vi "ASE Kalman_Experiment_FPGA.vi"() -> ()   [LabVIEW 2018]
doc: "This example demonstrates a simple analog loopback."
uses:
  <vilib>/Simulation/Scripting/Companion Diagram/SimConfigNode/SimParams.ctl
  <vilib>/Simulation/Scripting/Companion Diagram/SimConfigNode/_simSolvers.ctl
  <vilib>/Simulation/Implementation/Shared/SIMSCR Execution Mode.ctl
  <vilib>/Platform/TimedLoop/XDataNode/timing_clust.ctl
  <vilib>/Platform/TimedLoop/XDataNode/nitl_modes.ctl
  <vilib>/Platform/TimedLoop/XDataNode/wakeup.ctl
  <vilib>/Simulation/Param Hierarchy/Typedefs/SIMPH Param Control Actions.ctl
  <vilib>/addons/Control Design/_Stochastic Systems/Stochastic Systems.llb/Stochastic Systems SubVIs/cd_Second-Order Statistics Noise Model.ctl
  <vilib>/Simulation/Implementation/Shared/SIM limit type.ctl
  <vilib>/Simulation/Scripting/Editor Utilities/SIM subVI tag data.ctl
  <vilib>/Simulation/Scripting/Editor Utilities/SIM subVI execution type.ctl
  <vilib>/Simulation/Implementation/Shared/NILVSim_ParamChanged.vi
  <vilib>/Simulation/Implementation/Shared/NILVSim_FinishedLate.vi
  <vilib>/Simulation/Implementation/Shared/NILVSIM_BeginStep.vi
  <vilib>/Simulation/Utility/Implementation/SIM Halt.vi
  <vilib>/Simulation/DataSources/Implementation/NILVSim Signal Generator.llb/SIM Signal Generator (scalar).vi
  <vilib>/Simulation/Nonlinear/Implementation/NILVSim Saturation.llb/SIM Saturation (scalar).vi
  <vilib>/Simulation/ContinuousLinear/Implementation/NILVSim Integrator new.llb/SIM Integrator distributor (scalar).vi
  <vilib>/Simulation/ContinuousLinear/Implementation/NILVSim Integrator new.llb/SIM Integrator collector (scalar).vi
  <vilib>/Simulation/Utility/Implementation/NILVSim Memory.llb/NILVSim Memory (core).vi
  <vilib>/Simulation/ContinuousLinear/Implementation/NILVSim Transfer Function.llb/SIM Transfer Function Distributor (SISO).vi
  <vilib>/Simulation/SignalArithmetic/Implementation/NILVSim Gain.llb/SIM Gain (scalar).vi
  <vilib>/Simulation/ContinuousLinear/Implementation/NILVSim Transfer Function.llb/SIM Transfer Function Collector (SISO).vi
  <vilib>/Simulation/Nonlinear/Implementation/NILVSim RateLimiter.llb/SIM RateLimiter (scalar).vi
  <vilib>/Simulation/Implementation/Shared/SIM Fire Discrete SubVI.vi
  <vilib>/Simulation/Nonlinear/Implementation/NILVSim Saturation.llb/SIM Saturation (vector).vi
  <vilib>/Simulation/SignalArithmetic/Implementation/NILVSim Gain.llb/SIM Gain (vector).vi
  <vilib>/Simulation/SignalDisplay/Implementation/NILVSim Time Waveform.llb/SIM Time Waveform (vector).vi
  <vilib>/Simulation/Implementation/Shared/NILVSim_Manager.vi
  <vilib>/Utility/error.llb/Clear Errors.vi
  <vilib>/Simulation/Implementation/Shared/NILVSim_FinalizeModel.vi
  <vilib>/Simulation/Implementation/Shared/SIM Fire Discrete SubVI (Core).vi
  <vilib>/FPGAPlugInAG/cRIO-9068/niLvFpga_Open_cRIO-9068.vi
  <vilib>/rvi/interface/common/dynamic/niFpgaDynamicAddResources.vi
  <vilib>/imath/engines/lvmath2/RunTimeEngine/Managers/WorkSpace/UID Generator.vi
  <vilib>/imath/engines/lvmath2/RunTimeEngine/RunTimeType/NIMS_RunTimeType_From StrictType (excl LVString).vi
  <instcachedir>/0/NIMS_RunTimeType_From StrictType (excl LVString)_E7E34A65C99947108168652BAD14964D.lvgen/NIMS_RunTimeType_From StrictType (excl LVString)_E7E34A65C99947108168652BAD14964D_000.vi
  <vilib>/imath/engines/lvmath2/RunTimeEngine/LocalVariableDefStatement/MC_LocalVariableDefStatement_Display.vi
  <vilib>/imath/engines/lvmath2/RunTimeEngine/Managers/SymbolTable/Clear UID.vi
  <vilib>/imath/engines/lvmath2/RunTimeEngine/NodeEndStatement/NIMS_NodeEndStatement_Output.vi
  <instcachedir>/0/NIMS_NodeEndStatement_Output_53EC0D466D134D7ABD903AC30B43404B.lvgen/NIMS_NodeEndStatement_Output_53EC0D466D134D7ABD903AC30B43404B_010.vi
  <instcachedir>/0/NIMS_NodeEndStatement_Output_53EC0D466D134D7ABD903AC30B43404B.lvgen/NIMS_NodeEndStatement_Output_53EC0D466D134D7ABD903AC30B43404B_002.vi
  <vilib>/imath/engines/lvmath2/RunTimeEngine/ErrorHandling/NIMS_Finalize Error.vi
  <vilib>/addons/Control Design/_Stochastic Systems/Stochastic Systems.llb/CD Construct Stochastic Model (Numeric).vi
  <vilib>/addons/Control Design/_Stochastic Systems/Stochastic Systems.llb/CD Construct Noise Model (Numeric).vi
  <vilib>/Simulation/Implementation/Shared/SIM Unbundle Sim Info.vi
  <vilib>/Simulation/Implementation/Shared/SIMSH Read Queue.vi
  <vilib>/Simulation/Implementation/Shared/NILVSim_Initialize.vi
  <vilib>/Utility/error.llb/Error Cluster From Error Code.vi
  <vilib>/rvi/errors/niLvFpgaAdjustHostInterfaceError.vi
  <vilib>/Simulation/Utility/Implementation/NILVSim Get Time and IsAcceptedStep.vi
  <vilib>/Simulation/Implementation/Shared/NILVSim_GetModelError.vi
  <vilib>/Simulation/Implementation/Shared/SIM Bundle Sim Info.vi
  <vilib>/FPGAPlugInAG/Dynamic/niLvFpga_Close_Dynamic.vi
  <vilib>/rvi/interface/nirviOpenFPGA/nirviOpenFPGA.xnode
  FPGA Bitfiles/KalmanFilterASE_FPGATarget_FPGAQ1MODULE_8J-A6gSqyPk.lvbitx
  FPGA_Q1_MODULE.vi
  <vilib>/Simulation/Scripting/Companion Diagram/SimConfigNode/SimDog.xnode
  <vilib>/Quanser/Rapid Control Prototyping Toolkit/discrete/_TypeSpecific/CL Bias Removal (Scalar).vi
  <vilib>/Quanser/Rapid Control Prototyping Toolkit/discrete/CL Bias Removal.vi
  <vilib>/addons/Control Design/_Implementation/CD Continuous Recursive Kalman Filter.vi
  <vilib>/Platform/TimedLoop/XDataNode/XDataNode.xnode
  <vilib>/rvi/interface/nirviReadWriteControl/nirviReadWriteControl.xnode
  <vilib>/Simulation/Implementation/XNodeFramework/SimXNode/SimX.xnode
  <vilib>/rvi/interface/nirviCloseFPGA/nirviCloseFPGA.xnode
  <vilib>/Simulation/ContinuousLinear/Implementation/NILVSim Transfer Function.llb/SIM Transfer Function (SISO).vi
  <vilib>/Simulation/ContinuousLinear/Implementation/NILVSim Integrator new.llb/SIM Integrator (scalar).vi
  NiFpgaLv.dll
  <vilib>/rvi/interface/Simulation/niFpgaSimulationCallBeginRW.vi
  <vilib>/addons/Control Design/_Stochastic Systems/NI_CD_Stochastic Systems.lvlib
  <vilib>/imath/engines/lvmath2/RunTimeEngine/Managers/SymbolTable/NIMS_WorkSpace.lvlib
  <vilib>/Platform/TimedLoop/XDataNode/XDNodeRunTimeDep.lvlib
  <vilib>/Simulation/Implementation/Shared/NI_SIM_Implementation.lvlib
panel:
  out "Kalman Filter":waveform(dbl)[](graph)=[{"t0"=timestamp(9.964 s since 1904-01-01), "dt"=1.0, "Y"=[0.009999999999999988]}, {"t0"=timestamp(9.964 s since 1904-01-01), "dt"=1.0, "Y"=[0.008101035650175014]}, {"t0"=timestamp(9.964 s since 1904-01-01), "dt"=1.0, "Y"=[0.0033426903430059957]}]
  out "Measured value":T1(graph)={"output"=0.0096065956, "Result"=0.0090666584, "output"=0.0091514816}
  in  "R":dbl[][](array[numeric])=[[0.001, 0.0], [0.0, 0.001]] format="%#.5f"
  in  "Q":dbl[][](array[numeric])=[[0.001, 0.0, 0.0, 0.0], [0.0, 0.001, 0.0, 0.0], [0.0, 0.0, 0.001, 0.0], [0.0, 0.0, 0.0, 0.001]] format="%#.4f"
  in  "Enable Motor":bool
  in  "Setpoint Command":T2={"Amplitude (m)"=0.01, "Frequency (Hz)"=0.3} caption="Road (Bottom Plate)\nAmplitude Command (m)" {"Frequency (Hz)" min=0.0 max=0.5 step=0.009999999776482582 format="%_3f"; "Amplitude (m)" min=-10.0 max=10.0 step=0.5 format="%_3f"}
  in  "Halt?":bool
  # "Active Suspension Adaptive Control Experiment"
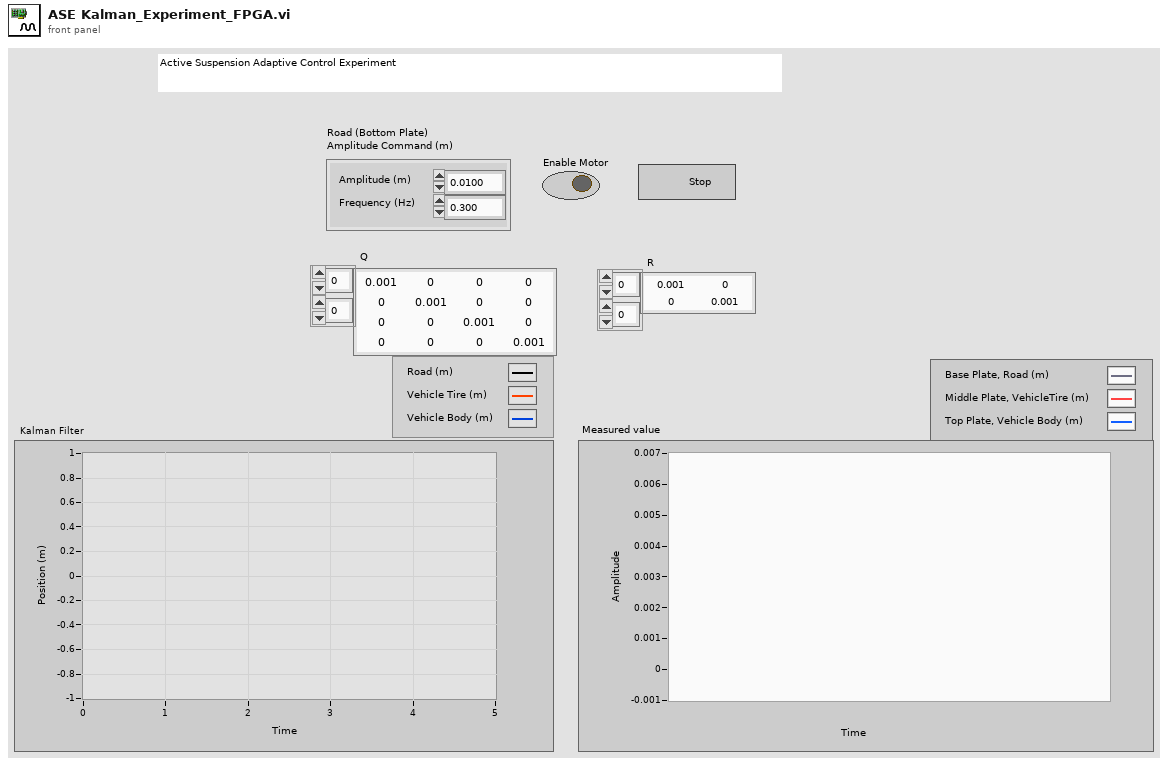
[diagram p1: front panel]
types:
  T1 = cluster{"output":dbl, "Result":dbl, "output":dbl}
  T2 = cluster{"Amplitude (m)":dbl, "Frequency (Hz)":dbl}
  T3 = typedef "SIMSCR Execution Mode.ctl" = enum16{"Simulate to Completion", "Single Time-Step Simulation (Fixed Step Only)"}
  T4 = typedef "XDNodeRunTimeDep.lvlib/timing_clust.ctl" = cluster{"Expected End [f-1]":u64, "Actual End [f-1]":u64, "Finished Late? [f-1]":bool, "Expected End [i-1]":u64, "Actual End [i-1]":u64, "Finished Late? [i-1]":bool, "Expected Start [i]":u64, "Actual Start [i]":u64, "Expected Start [f]":u64, "Actual Start [f]":u64, "Source Name":string, "Structure Name":string, "Period":i64, "Deadline":i64, "Offset":i64, "Start":i64, "Priority":i32, "Timeout":i32, "Mode":T5, "Wakeup Reason":T6, "Error":errorcluster, "Source Type":string, "Secondary Source Type":string, "Global End Time":u64, "Global Start Time":u64, "Frame Duration":u64, "Iteration Duration":u64, "Assigned CPU":i32, "I/O Scan Engine Mode":u32}
  T5 = typedef "XDNodeRunTimeDep.lvlib/nitl_modes.ctl" = enum32{"No Change", "Process missed periods, maintain original phase", "Discard missed periods, maintain original phase", "Process missed periods, ignore original phase", "Discard missed periods, ignore original phase"}
  T6 = typedef "XDNodeRunTimeDep.lvlib/wakeup.ctl" = enum32{"Normal", "Aborted", "Asynchronous wakeup", "Timing source error", "Timed loop error", "Timeout"}
  T7 = typedef "SIMPH Param Control Actions.ctl" = enum16{"get params", "set params"}
  T8 = typedef "SIM subVI tag data.ctl" = cluster{"period":dbl, "skew":dbl, "Simulation execution type":T9}
  T9 = typedef "SIM subVI execution type.ctl" = enum16{"Function call", "Discrete", "Continuous", "Initialization only", "Final step only"}
  T10 = typedef "SIM limit type.ctl" = enum16{"upper", "lower", "both", "none"}
  T11 = cluster{"SIMSH Sim Time":dbl, "CL Enabled Moving Average (Scalar)":cluster{"output":dbl}, "CL Enabled Moving Average (Scalar) - SIMSH":cluster{"SIMSH Sim Time":dbl, "Memory 2":cluster{"output":dbl[]}, "states on enable":enum16{"reset average", "cumulative average"}, "Select 2":cluster{"s? t:f":dbl}, "Memory":cluster{"output":dbl}, "Index Array 2":cluster{"element":dbl}, "Divide 2":cluster{"x/y":dbl}, "Select":cluster{"s? t:f":dbl[]}, "Summation":cluster{"Result":dbl[]}, "Discrete Delay":cluster{"output":dbl[]}, "Not":cluster{".not. x?":bool}, "Initialize Array 3":cluster{"initialized array":dbl[]}, "Array Size 2":cluster{"size(s)":i32}, "Build Array":cluster{"appended array":dbl[]}}, "initial value":dbl, "Select":cluster{"s? t:f":dbl}, "Not":cluster{".not. x?":bool}, "Subtract":cluster{"x-y":dbl}, "And":cluster{"x .and. y?":bool}, "Less?":cluster{"x < y?":bool}, "Greater Or Equal?":cluster{"x >= y?":bool}, "Simulation Time":cluster{"simulation time":dbl}}
  T12 = typedef "NI_CD_Stochastic Systems.lvlib/cd_Second-Order Statistics Noise Model.ctl" = cluster{"Q":dbl[][], "E{w}":dbl[], "E{v}":dbl[], "R":dbl[][], "N":dbl[][]}
  T13 = cluster{"Sampling Time (s)":dbl, "G":dbl[][], "B":dbl[][], "A":dbl[][], "C":dbl[][], "D":dbl[][], "H":dbl[][]}
  T14 = cluster{"SIMSH Sim Time":dbl, "Subsystem":cluster{"A(t)":dbl[][]}, "Subsystem - SIMSH":cluster{"SIMSH Sim Time":dbl, "Integrator":cluster{"output":dbl[]}, "sym matrix to compact form.vi":cluster{"Compact Form":dbl[]}, "sym matrix to compact form.vi 2":cluster{"Compact Form":dbl[]}, "compact form to sym matrix.vi":cluster{"Symmetric Matrix":dbl[][]}, "Pre-allocated 0_nxn":dbl[][]}, "Integrator":cluster{"output":dbl[]}, "cd_Adjust Model for Non-Zero-Mean Noise_No_Case.vi":cluster{"B(k) out":dbl[][], "D(k) out":dbl[][], "u(k) out":dbl[], "y(k) out":dbl[]}, "Unbundle By Name 3":cluster{"E{w(t)}=0?":bool, "E{v(t)}=0?":bool}, "Unbundle By Name 2":cluster{"P(0) out":dbl[][], "xhat(0) out":dbl[]}, "Unbundle By Name":cluster{"E{w}":dbl[], "E{v}":dbl[], "Q":dbl[][], "R":dbl[][], "N":dbl[][]}, "cd_Calculate Continuous Recursive Kalman Filter Gain.vi":cluster{"L(t)":dbl[][], "error out":errorcluster}, "cd_Differential Riccati Equation Point-by-Point.vi":cluster{"d[P(t)]/dt":dbl[][], "error out":errorcluster}, "cd_Continuous Recursive Kalman Filter Point-by-Point.vi":cluster{"d[xhat(t)]/dt":dbl[], "yhat(t)":dbl[], "error out":errorcluster}, "cd_Check Models Change for Continuous Recurisve Kalman Filter.vi":cluster{"0_qxm":dbl[][], "0_nxm":dbl[][], "0_nx1":dbl[], "0_nxq":dbl[][], "0_mx1":dbl[], "0_mxq":dbl[][], "0_mxn":dbl[][], "Identitiy nxn":dbl[][], "xhat(0) and P(0)":cluster{"xhat(0) out":dbl[], "P(0) out":dbl[][]}, "0_mxm":dbl[][], "E{w} and E{v}=0?":cluster{"E{w(t)}=0?":bool, "E{v(t)}=0?":bool}, "0_nxn":dbl[][], "0_m(m+1)/2":dbl[], "A":dbl[][], "B":dbl[][], "G":dbl[][], "C":dbl[][], "D":dbl[][], "H":dbl[][], "Second-Order Statistics Noise Model Out":cluster{"Q":dbl[][], "E{w}":dbl[], "E{v}":dbl[], "R":dbl[][], "N":dbl[][]}, "0_n(n+1)/2":dbl[]}}
  T15 = typedef "SimParams.ctl" = cluster{"Initial Time (s)":dbl, "Final Time (s)":dbl, "Step Size (s)":dbl, "ODE Solver":T16, "Minimum Step Size (s)":dbl, "Maximum Step Size (s)":dbl, "Relative Tolerance":dbl, "Absolute Tolerance":dbl, "Software Timing":bool, "Initial Step Size (s)":dbl, "Automatic Fixed Step Size?":bool, "Automatic Discrete Step Size?":bool, "Discrete Step Size (s)":dbl, "Calculate using Time Step":bool, "Solver Wired?":bool, "Prev.Frm.Expected End":u64, "Prev.Frm.Actual End":u64, "Prev.Frm.Finished Late?":bool, "Prev.Iter.Expected End":u64, "Prev.Iter.Actual End":u64, "Prev.Iter.Finished Late?":bool, "Expected Iteration Start":u64, "Actual Iteration Start":u64, "Expected Frame Start":u64, "Actual Frame Start":u64, "Source Name":string, "Name":string, "Period":i64, "Deadline":i64, "Offset":i64, "Start":i64, "Priority":i32, "Timeout":i32, "Processor":i32, "Mode":enum32{"No Change", "Process missed periods, maintain original phase", "Discard missed periods, maintain original phase", "Process missed periods, ignore original phase", "Discard missed periods, ignore original phase"}, "Wakeup reason":enum32{"Normal", "Aborted", "Asynchronous wakeup", "Timing source error", "Timed loop error", "Timeout"}, "Error":errorcluster, "Source Type":string, "Secondary Source Type":string, "Global End Time":u64, "Global Start Time":u64, "Full Solver Reset":bool, "Execution Mode":T3, "Nan/Inf Check":bool, "Custom Solver Library":string, "Solver Is Variable":bool, "custom solver name":string, "Signal Collection Decimation":u32}
  T16 = typedef "_simSolvers.ctl" = enum16{"Runge-Kutta 1 (Euler)", "Runge-Kutta 2", "Runge-Kutta 3", "Runge-Kutta 4", "Runge-Kutta 23 (variable)", "Runge-Kutta 45 (variable)", "BDF (variable)", "Adams-Moulton (variable)", "Rosenbrock (variable)", "Discrete States Only", "SDIRK 4 (variable)", "Radau 5 (variable)", "Radau 9 (variable)", "Radau 13 (variable)", "Radau [Variable Order] (variable)", "Gear's Method (variable)", "Linearizer", "State Query", "Trim Eval", "Custom Solver"}
  T17 = typedef "NI_CD_Stochastic Systems.lvlib/cd_Stochastic State-Space Model.ctl" = cluster{"Sampling Time (s)":dbl, "G":dbl[][], "B":dbl[][], "A":dbl[][], "C":dbl[][], "D":dbl[][], "H":dbl[][]}
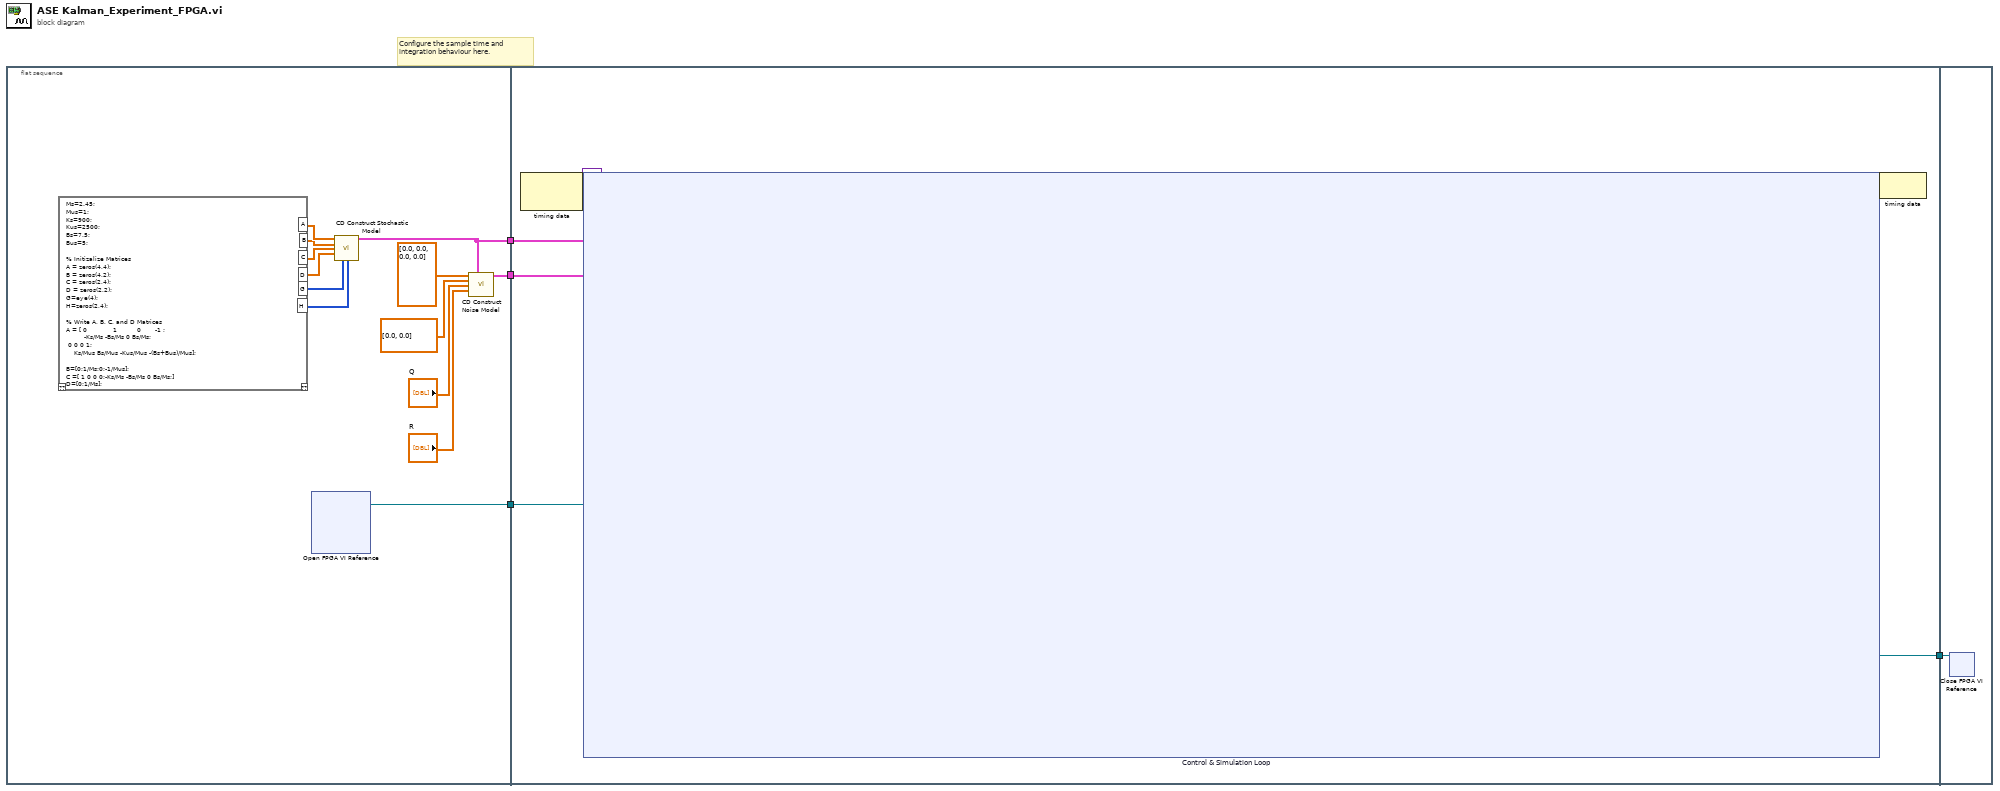
[diagram p0: block diagram]
diagram:
  # "Configure the sample time and integration behaviour here."
  n1 = flat-sequence {
    tunnel: [w17] -> w4
    tunnel: [w6] -> w2
    tunnel: [w5] -> w1
    tunnel: w4 -> [w207]
    tunnel: [w208] -> w3
    tunnel: w2 -> [w206]
    tunnel: w1 -> [w205]
    tunnel: w3 -> [w1322]
    frame #0 {
      n2 = mathscript code="Ms=2.45;\nMus=1;\nKs=900;\nKus=2500;\nBs=7.5;\nBus=5;\n\n% Initizalize Matrices\nA = zeros(4,4);\nB = zeros(4,2);\nC = zeros(2,4);\nD = zeros(2,2);\nG=eye(4);\nH=zeros(2,4);\n\n% Write A, B, C, and D Matrices\nA = [ 0             1          0       -1 ; \n         -Ks/Ms -Bs/Ms 0 Bs/Ms;  \n 0 0 0 1;\n    Ks/Mus Bs/Mus -Kus/Mus -(Bs+Bus)/Mus];\n\nB=[0;1/Ms;0;-1/Mus];\nC =[ 1 0 0 0;-Ks/Ms -Bs/Ms 0 Bs/Ms;]\nD=[0;1/Ms];"() -> ("A"=w16:dbl[][], "B"=w14:dbl[][], "C"=w15:dbl[][], "D"=w13:dbl[][], "G"=w10:i32[][], "H"=w9:i32[][])  [unwired: 1 in, 1 out]
      n3 = xnode "Open FPGA VI Reference"() -> ("FPGA VI Reference Out"=w17:refnum<k20>)  [unwired: 2 in, 1 out]
      n4 = call-poly <vilib>:"CD Construct Stochastic Model.vi"("A"=w16, "B"=w14, "C"=w15, "D"=w13, "G"=w10, "H"=w9) -> ("Stochastic State-Space Model"=w6:T17)  [unwired: 2 in, 7 out]
      n5 = call-poly <vilib>:"CD Construct Noise Model.vi"("E{w}"=dbl[] [0.0, 0.0, 0.0, 0.0], "Stochastic State-Space Model"=w6, "E{v}"=dbl[] [0.0, 0.0], "Q"="Q", "R"="R") -> ("Second-Order Statistics Noise Model out"=w5:T12)  [unwired: 9 in, 1 out]
    }
    frame #1 {
      n6 = node-c288() -> (w210:variant)  [unwired: 2 in]
      n7 = node-c254 "Control & Simulation Loop"(w210, w207, w206, w205) -> (w209:variant, w208:refnum<k20>)
      n8 = node-c288(w209) -> ()  [unwired: 1 out]
    }
    frame #2 {
      n9 = xnode "Close FPGA VI Reference"("FPGA VI Reference In"=w1322) -> ()  [unwired: 1 in, 1 out]
    }
  }
